vi "4Pi 4Pi Modes - Mode Scan Engine.vi"() -> ()   [LabVIEW 2016]
uses:
  4Pi 4Pi Modes - Controls/4Pi 4Pi Modes - Mode Scan - Gaussian Initial Guesses.ctl
  4Pi 4Pi Modes - Controls/4Pi 4Pi Modes - Mode Scan - Metric Fit Type.ctl
  4Pi 4Pi Modes - Controls/4Pi 4Pi Modes - Mode Scan - Scan Settings.ctl
  4Pi 4Pi Modes - Controls/4Pi 4Pi Modes - Mode Scan - Metric.ctl
  4Pi 4Pi Modes - Controls/4Pi 4Pi Modes - Mode Scan - Threshold Mean Limits.ctl
  4Pi 4Pi Modes - Controls/4Pi 4Pi Modes - Mode Scan - Image Type.ctl
  4Pi 4Pi Modes - Controls/4Pi 4Pi Modes - Mode Scan - Blink Scan Settings.ctl
  4Pi 4Pi Modes - Controls/4Pi 4Pi Modes - Mode Scan - Blink Analysis Type.ctl
  <vilib>/vision/Image Controls.llb/IMAQ Image.ctl
  Hardware Configuration/Hardware Configuration Controls/Device Type.ctl
  Hardware Configuration/Hardware Configuration Controls/Device Function.ctl
  <vilib>/Utility/miscctls.llb/LVPointTypeDef.ctl
  4Pi 4Pi Modes - Controls/4Pi 4Pi Modes - Mode Scan - Last Used Data Type.ctl
  4Pi 4Pi Modes - Controls/4Pi 4Pi Modes - Mode Scan - Notifier Type.ctl
  4Pi 4Pi Modes - Controls/4Pi 4Pi Modes - Mode Scan - Scan Actions.ctl
  4Pi 4Pi Modes - Controls/4Pi 4Pi Modes - Standard Action.ctl
  4Pi 4Pi Modes - Controls/4Pi 4Pi Modes - Standard Counter Action.ctl
  <vilib>/Analysis/6fits.llb/Curve Fitting Criteria.ctl
  <vilib>/Analysis/baseanly.llb/Mean (DBL).vi
  <vilib>/Analysis/NI_AALBase.lvlib
  <vilib>/Analysis/NI_AALPro.lvlib
  <vilib>/gmath/NI_Gmath.lvlib
  <resource>/objmgr/IMAQImage.rc
panel:
  in  "Calling VI Ref":refnum<vi>
  in  "Main Tab":enum32{"Scan Modes", "Settings"}(tab)
  in  "Fit Data":bool
  in  "Apply":bool
  in  "Get Image":bool
  in  "Current Mode":i32(ring) items=["1", "2", "3", "4", "5", "6", "7", "8", "9", "10", "11", "12", "13", "14", "15", "16", "17", "18", "19", "20", "21", "22", "23", "24", "25", "26", "27", "28", "29", "30", "31", "32", "33", "34", "35", "36", "37", "38", "39", "40", "41", "42", "43", "44", "45", "46", "47", "48", "49", "50", "51", "52", "53", "54", "55", "56", "57", "58", "59", "60", "61", "62", "63", "64", "65", "66", "67", "68", "69", "70", "71", "72", "73", "74", "75", "76", "77", "78", "79", "80", "81", "82", "83", "84", "85", "86", "87", "88", "89", "90", "91", "92", "93", "94", "95", "96", "97", "98", "99", "100", "101", "102", "103", "104", "105", "106", "107", "108", "109", "110", "111", "112", "113", "114", "115", "116", "117", "118", "119", "120", "121", "122", "123", "124", "125", "126", "127", "128", "129", "130", "131", "132", "133", "134", "135", "136", "137", "138", "139", "140"]
  in  "Scan Mode":bool
  in  "Scan Next Mode":bool
  in  "Auto Scan Modes":bool
  out "Metric":cluster{dbl[], dbl[]}[](graph)
  out "AO Image Display":T1(plugin-control)
  in  "Gaussian Initial Guesses":T2={"Amplitude"=2500.0, "Center Position"=0.0, "Width (Sigma)"=200.0, "Offset"=500.0, "User Guesses"=TRUE}
  in  "DM Scan Settings":T3={"Frame Delay"=1, "Frame Accumulations"=2, "Number of Steps"=8, "Step Size (nm)"=80}
  in  "Image Type":T4 items=["Full Image", "ROI", "Blinks"]
  in  "Image Selection":i32(ring) items=["Quad 01", "Quad 02", "Quad 03", "Quad 04"]
  in  "Metric":T5=1 items=["Max Intensity", "No Zero Mean", "Threshold Mean", "Mean"]
  in  "Metric Fit Type":T6 items=["Guassian", "Quadratic"]
  in  "Threshold Mean Limits":T7={"Upper Limit"=10000.0, "Lower Limit"=0.0}
  in  "Blink Scan Settings":T8={"Blink Analysis Type"=1, "Blink ROI Box Width"=0, "Blink Threshold"=0.0} {"Blink Analysis Type" items=["Mean Intensity", "2D Fit Intensity"]}
  in  "Exit":bool
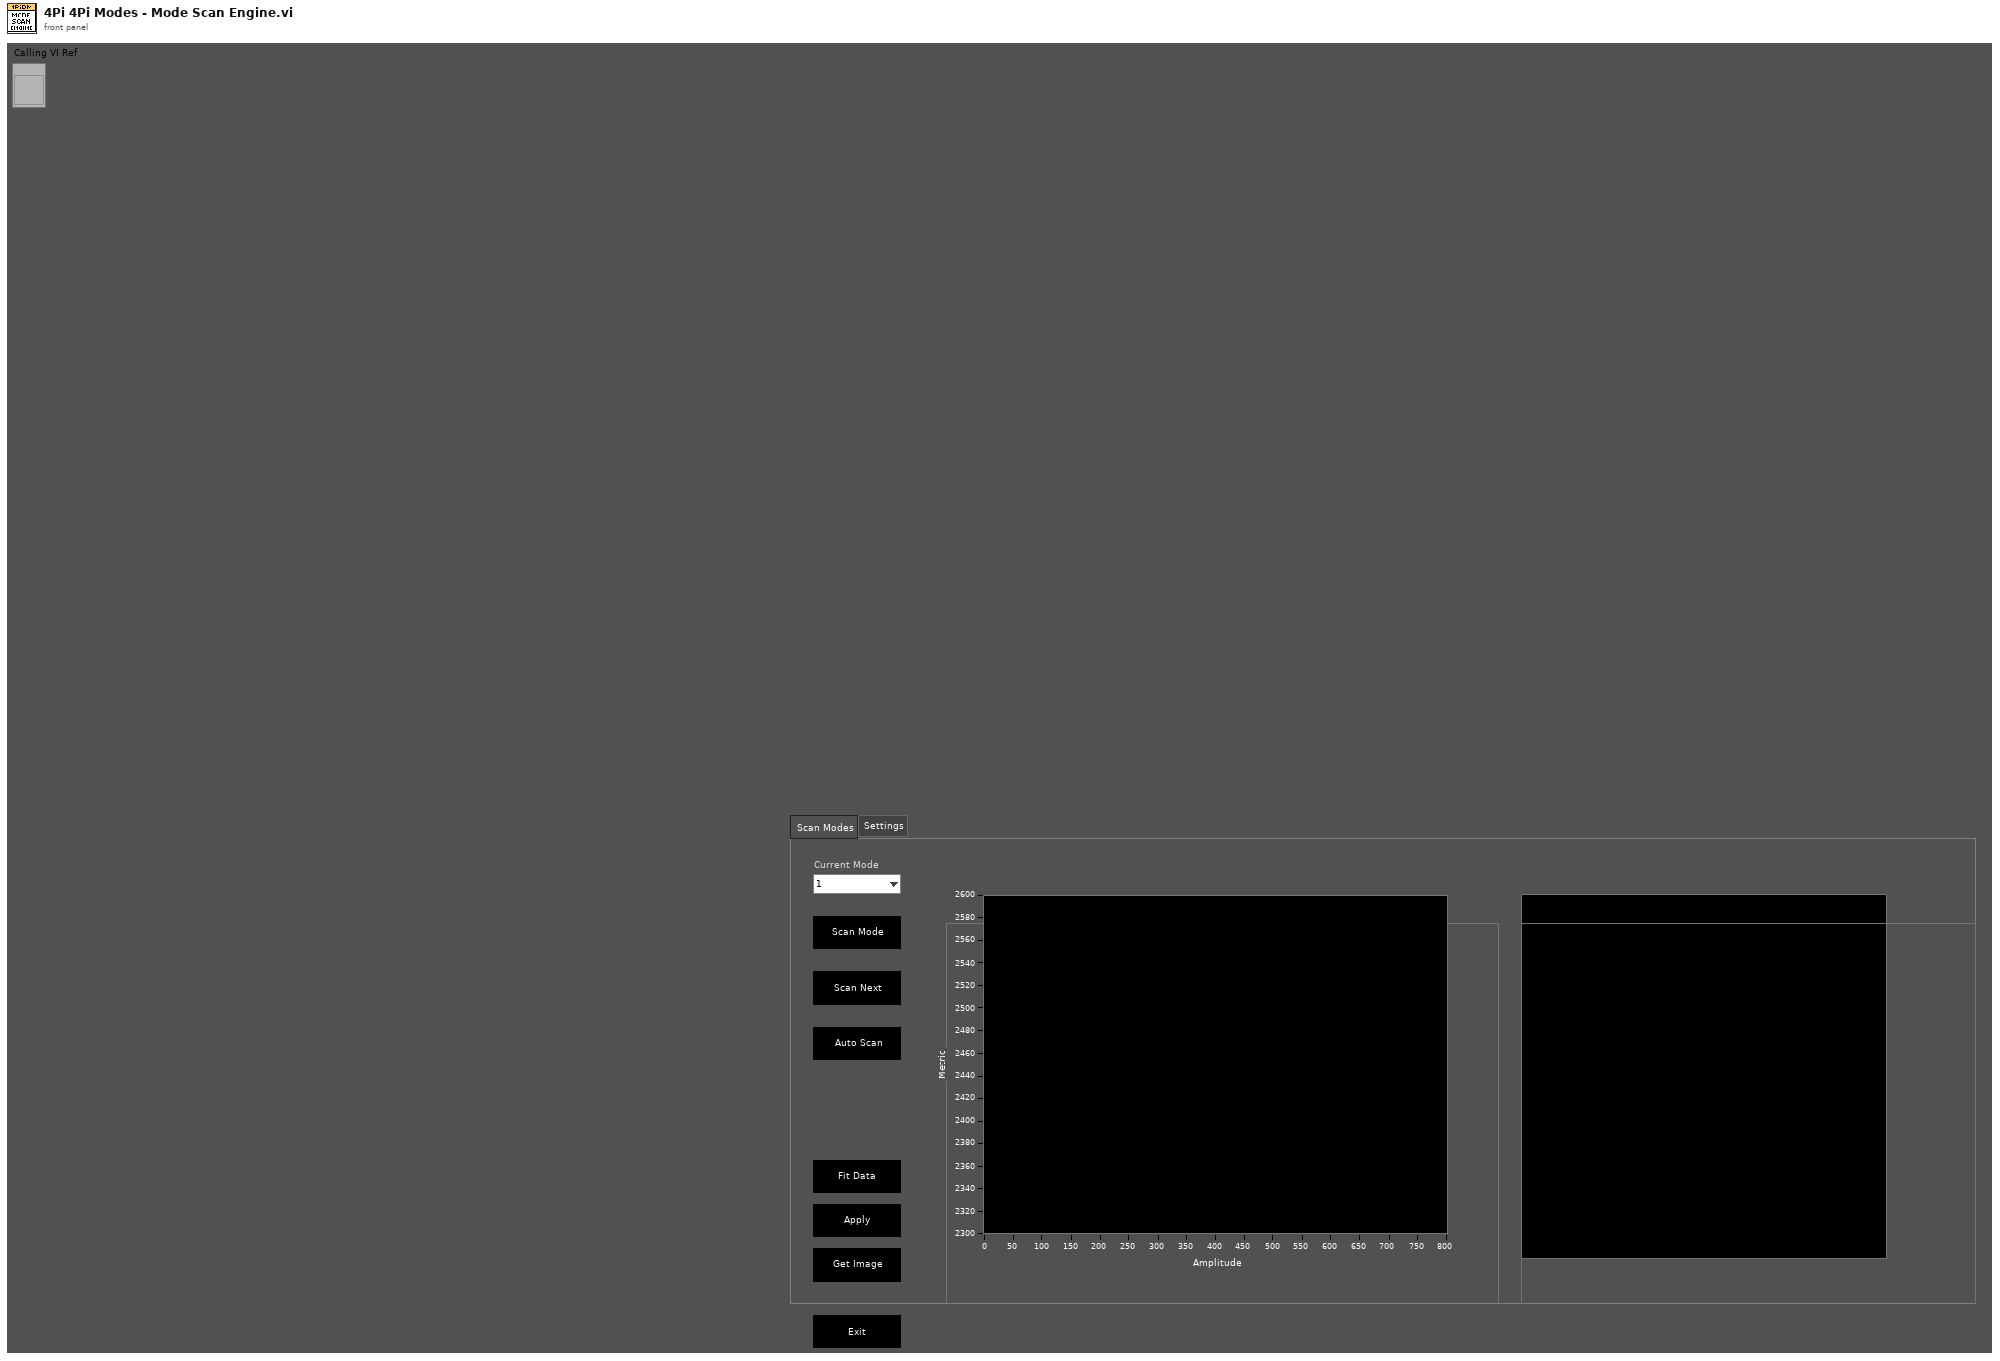
[diagram p1: front panel]
types:
  T1 = typedef "IMAQ Image.ctl" = refnum<image>
  T2 = typedef "4Pi 4Pi Modes - Mode Scan - Gaussian Initial Guesses.ctl" = cluster{"Amplitude":dbl, "Center Position":dbl, "Width (Sigma)":dbl, "Offset":dbl, "User Guesses":bool}
  T3 = typedef "4Pi 4Pi Modes - Mode Scan - Scan Settings.ctl" = cluster{"Frame Delay":u32, "Frame Accumulations":u16, "Number of Steps":u16, "Step Size (nm)":u16}
  T4 = typedef "4Pi 4Pi Modes - Mode Scan - Image Type.ctl" = u16
  T5 = typedef "4Pi 4Pi Modes - Mode Scan - Metric.ctl" = u16
  T6 = typedef "4Pi 4Pi Modes - Mode Scan - Metric Fit Type.ctl" = u16
  T7 = typedef "4Pi 4Pi Modes - Mode Scan - Threshold Mean Limits.ctl" = cluster{"Upper Limit":dbl, "Lower Limit":dbl}
  T8 = typedef "4Pi 4Pi Modes - Mode Scan - Blink Scan Settings.ctl" = cluster{"Blink Analysis Type":T9, "Blink ROI Box Width":u8, "Blink Threshold":sgl}
  T9 = typedef "4Pi 4Pi Modes - Mode Scan - Blink Analysis Type.ctl" = u16
  T10 = typedef "Image Type" = u32
  T11 = enum8{"Enabled", "Disabled", "Disabled and Grayed Out"}
  T12 = typedef "4Pi 4Pi Modes - Mode Scan - Scan Actions.ctl" = enum16{"Scan Mode", "Fit Data", "Scan Next Mode", "Update Mode Amount", "Get Image", "Compute Metric", "Update Counter", "Apply Correction", "Exit", "Quit"}
  T13 = typedef "4Pi 4Pi Modes - Mode Scan - Notifier Type.ctl" = cluster{"Action":T12, "Image Ref":T1, "Image Type":T4, "Fit Type":T6, "Metric":T5, "Scan Running?":bool, "DM Scan Settings":T3, "Threshold Mean Limits":T7, "Gaussian Initial Guesses":T2, "Blink Scan Settings":T8}
  T14 = typedef "4Pi 4Pi Modes - Mode Scan - Last Used Data Type.ctl" = cluster{"Image Ref Index":i32, "Image Type":T4, "Fit Type":T6, "Metric":T5, "DM Scan Settings":T3, "Threshold Mean Limits":T7, "Gaussian Initial Guesses":T2, "Blink Scan Settings":T8}
  T15 = enum16{"Always On", "Always Off", "Off While Running"}
  T16 = typedef "LVPointTypeDef.ctl" = cluster{"Horizontal":i16, "Vertical":i16}
  T17 = typedef "Device Function.ctl" = enum16{"Primary", "Secondary", "Overview", "Wide Field Drift Correction", "642 nm Excitation", "560 nm Excitation", "940 nm Excitation", "546 nm Excitation", "488 nm Excitation", "405 nm Excitation", "Objective Drift Correction", "4Pi Objective Lock", "Objective XY", "Objective Z", "Sample XY", "Sample Coarse Z", "Sample Z", "4Pi Lower", "4Pi Upper", "Mojo", "Adj Cavity", "Line Scanning", "Alert"}
  T18 = typedef "Device Type.ctl" = enum16{"AOTF", "Camera", "Deformable Mirror", "Laser", "Shutter", "Stage", "Waveform", "FPGA", "Email"}
  T19 = typedef "LVRectTypeDef.ctl" = cluster{"Left":i16, "Top":i16, "Right":i16, "Bottom":i16}
  T20 = typedef "LVBoundsTypeDef.ctl" = cluster{"Width":u32, "Height":u32}
  T21 = typedef "4Pi 4Pi Modes - Standard Action.ctl" = enum16{"Read", "Write"}
  T22 = typedef "4Pi 4Pi Modes - Standard Counter Action.ctl" = enum16{"Initialize", "Update Count", "Get Count"}
  T23 = cluster{"initial amplitude":dbl, "initial center":dbl, "initial standard deviation":dbl, "offset":dbl}
  T24 = cluster{"amp min":dbl, "amp max":dbl, "center min":dbl, "center max":dbl, "deviation min":dbl, "deviation max":dbl, "offset min":dbl, "offset max":dbl}
  T25 = enum16{"Linear", "Polynomial", "Exponential", "Power"}
  T26 = cluster{"Global Rectangle":i32[], "Contours":cluster{"Contour Type":u32, "ROI Type":u32, "Points":i32[]}[]}
  T27 = cluster{"Amplitude Out":dbl[], "Metric Out":dbl[]}
  T28 = cluster{"initial amplitude":dbl, "Numeric":dbl, "initial standard deviation":dbl, "offset":dbl}
  T29 = typedef "NI_AALPro.lvlib/Curve Fitting Criteria.ctl" = u16
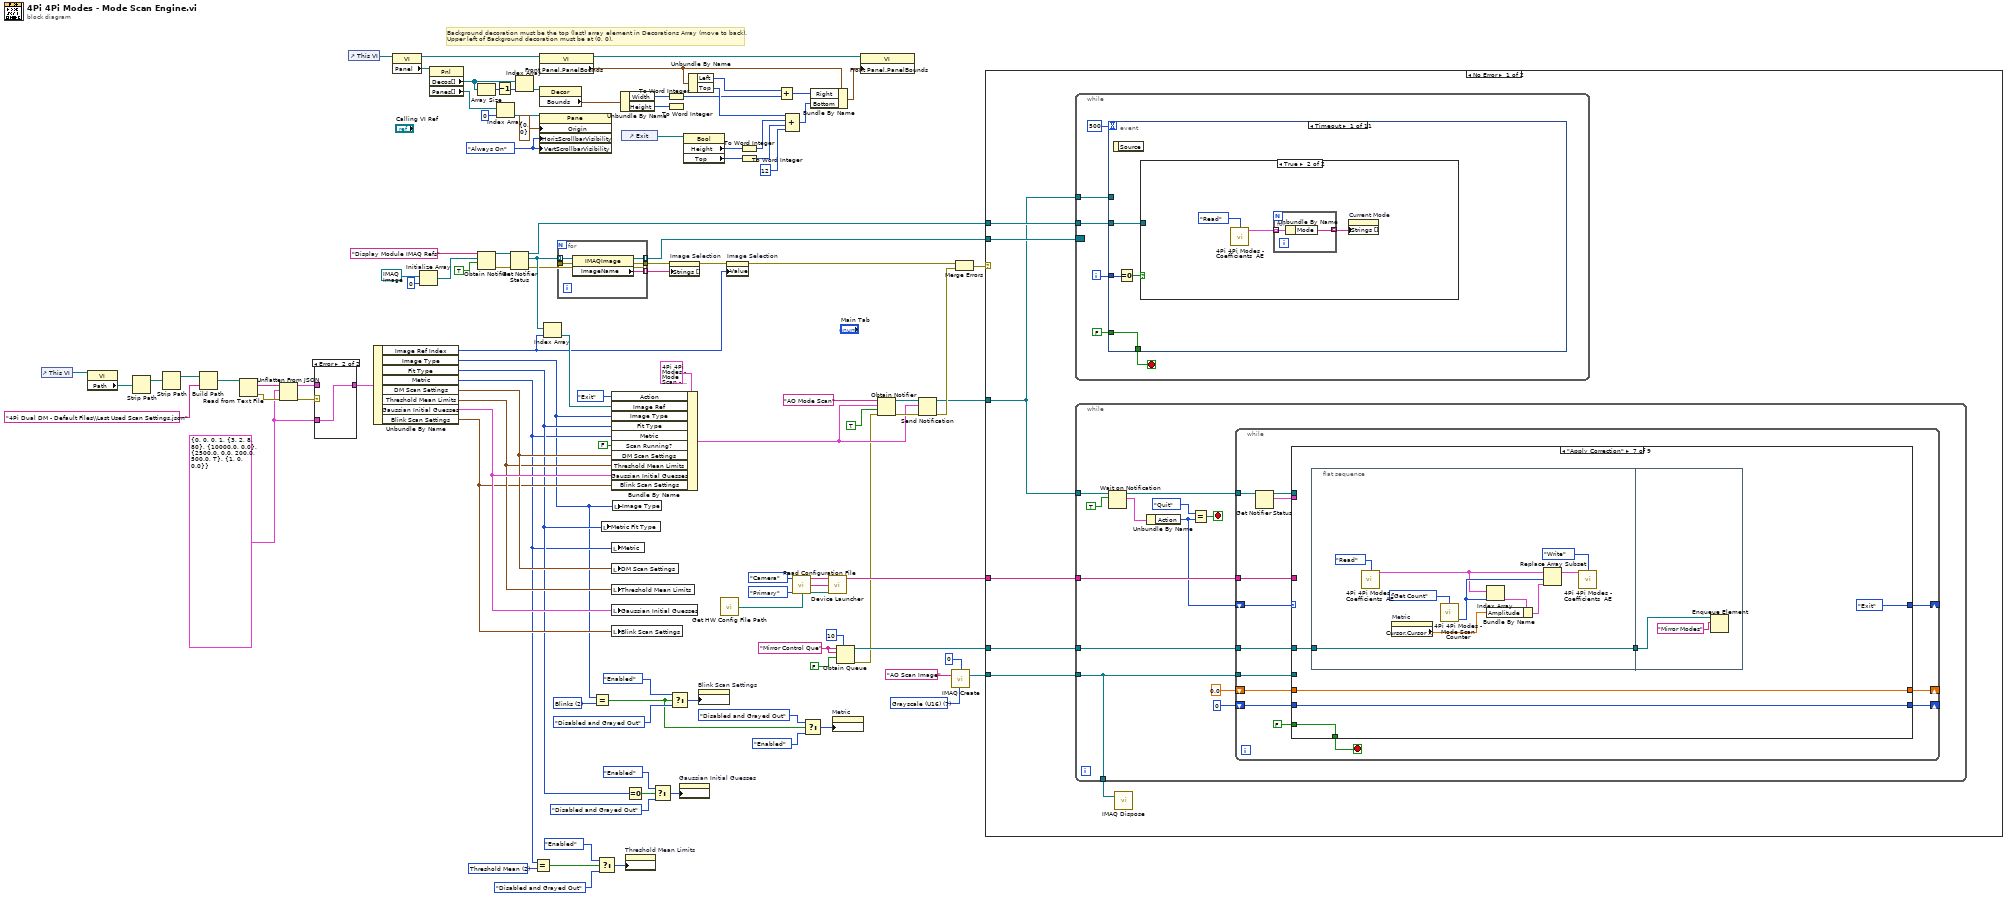
[diagram p0: block diagram]
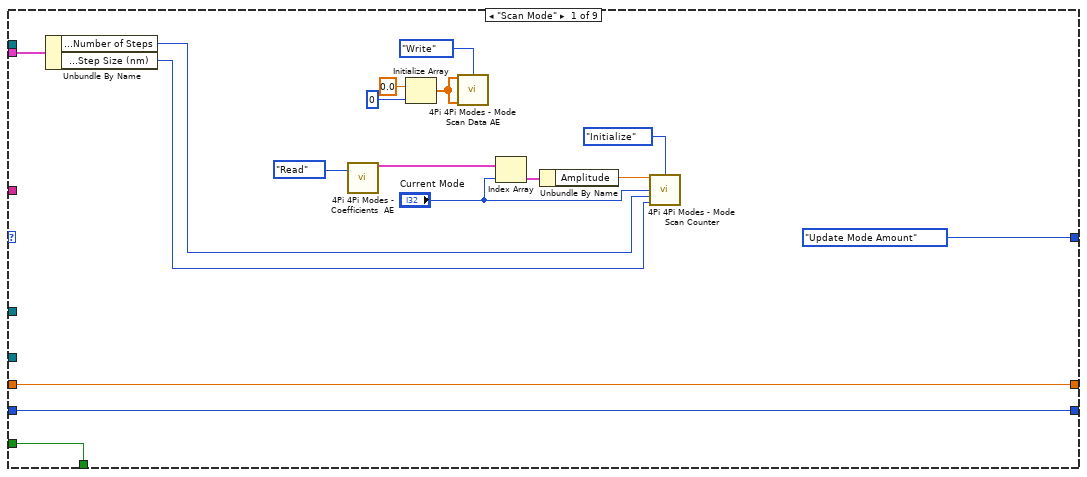
[diagram p2: hidden frame]
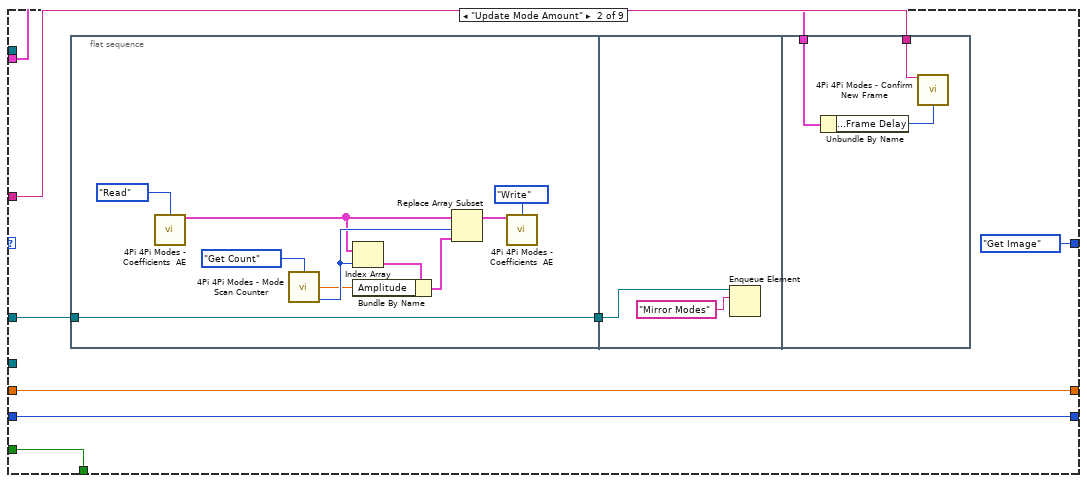
[diagram p3: hidden frame]
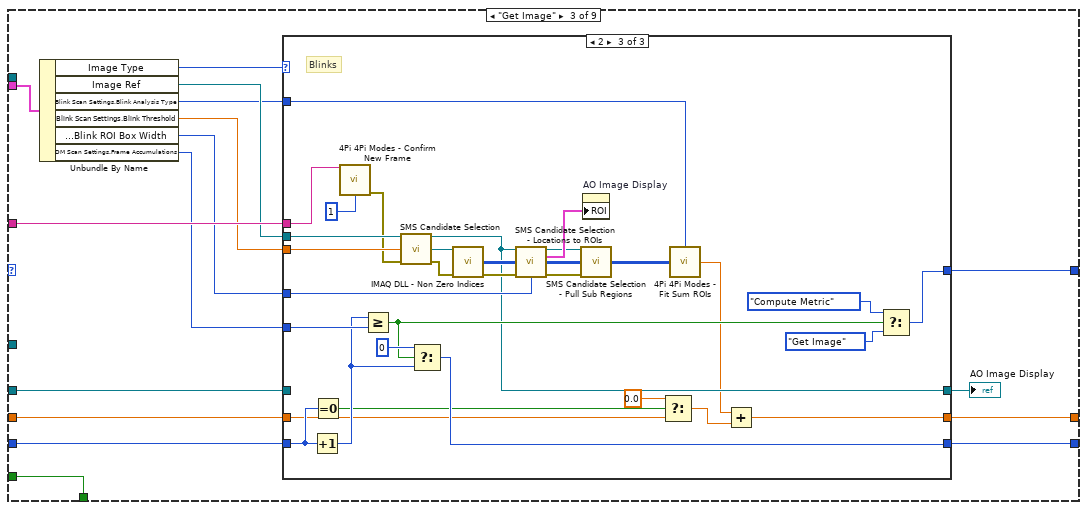
[diagram p4: hidden frame]
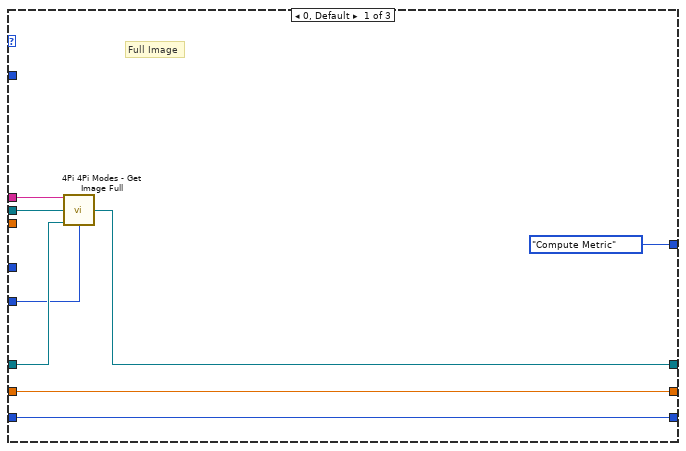
[diagram p5: hidden frame]
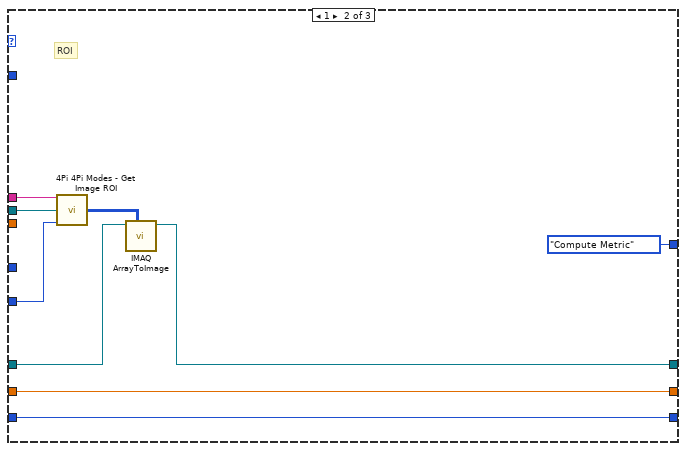
[diagram p6: hidden frame]
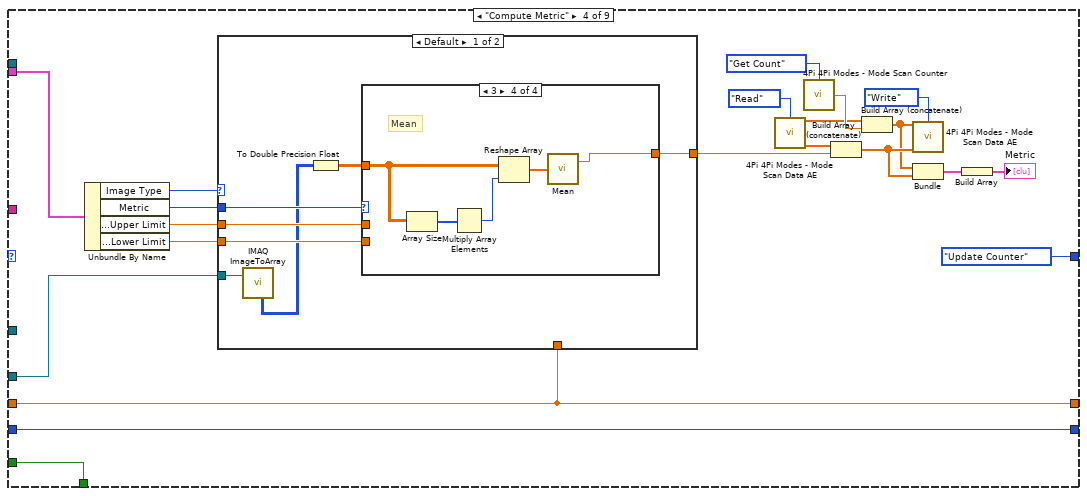
[diagram p7: hidden frame]
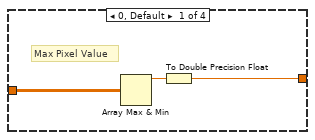
[diagram p8: hidden frame]
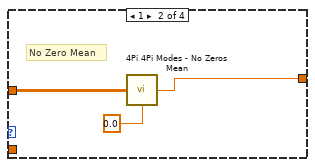
[diagram p9: hidden frame]
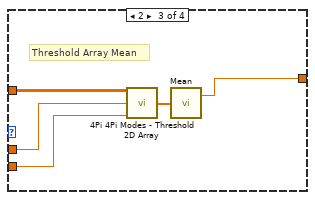
[diagram p10: hidden frame]
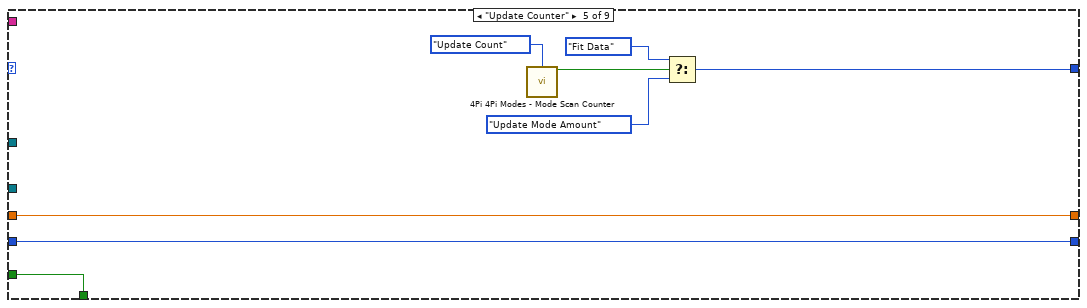
[diagram p12: hidden frame]
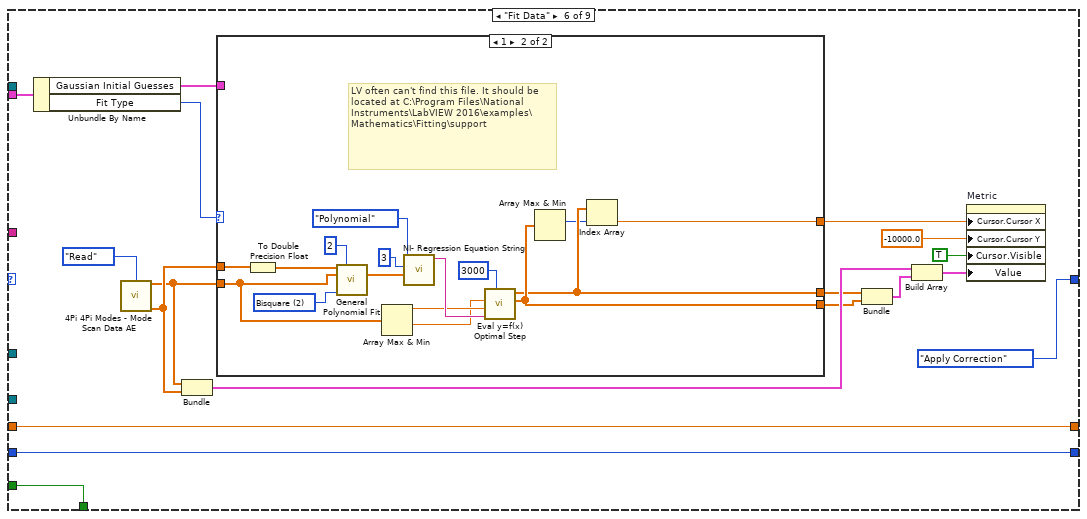
[diagram p13: hidden frame]
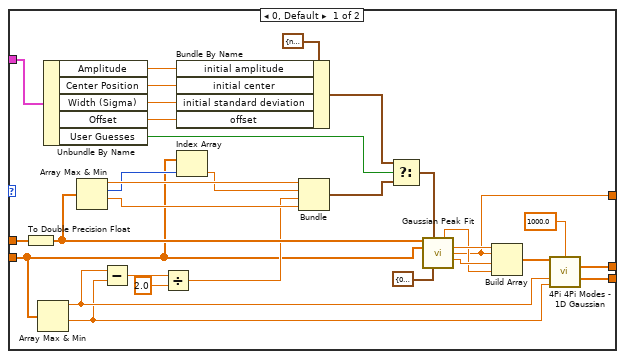
[diagram p14: hidden frame]
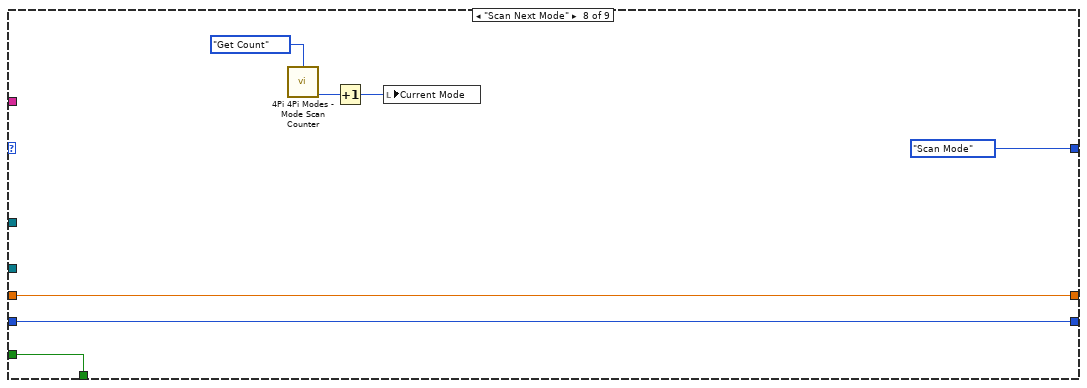
[diagram p15: hidden frame]
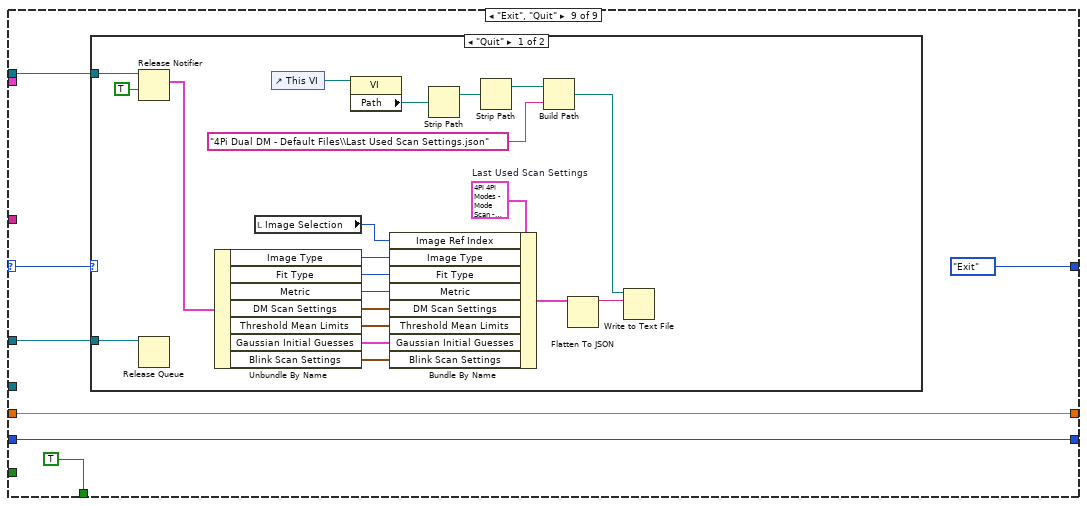
[diagram p16: hidden frame]
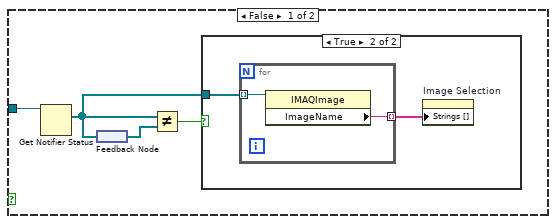
[diagram p18: hidden frame]
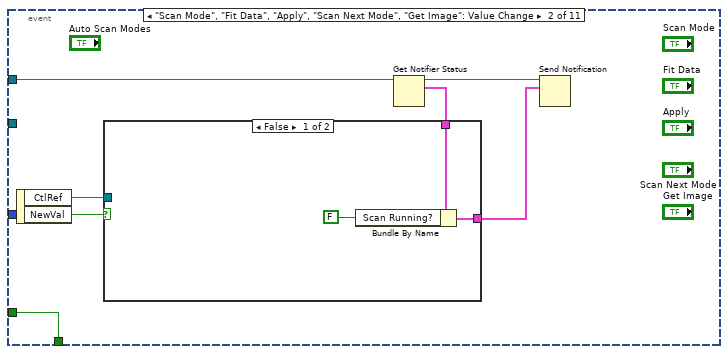
[diagram p20: hidden frame]
diagram:
  w2 = T10 7 items=["Grayscale (U8)", "Grayscale (I16)", "Grayscale (SGL)", "Complex (CSG)", "RGB (U32)", "HSL (U32)", "RGB (U64)", "Grayscale (U16)"] ("Image Type")
  w12 = T4 2 items=["Full Image", "ROI", "Blinks"] ("y")
  w15 = T5 2 items=["Max Intensity", "No Zero Mean", "Threshold Mean", "Mean"] ("y")
  w45 = T14 {"Image Ref Index"=0, "Image Type"=0, "Fit Type"=0, "Metric"=1, "DM Scan Settings"={"Frame Delay"=3, "Frame Accumulations"=2, "Number of Steps"=8, "Step Size (nm)"=80}, "Threshold Mean Limits"={"Upper Limit"=10000.0, "Lower Limit"=0.0}, "Gaussian Initial Guesses"={"Amplitude"=2500.0, "Center Position"=0.0, "Width (Sigma)"=200.0, "Offset"=500.0, "User Guesses"=TRUE}, "Blink Scan Settings"={"Blink Analysis Type"=1, "Blink ROI Box Width"=0, "Blink Threshold"=0.0}} ("Mode Scan Notifier Type")
  w76 = T15."Always On" ("Vertical Scrollbar Visibility")
  w109 = "Mirror Control Que" ("name (unnamed)")
  # "Background decoration must be the top (last) array element in Decorations Array (move to back).\nUpper left of Background decoration must be at (0, 0)."
  n1 = control-ref of="This VI"() -> (w58:refnum<vi>)
  n2 = property class="VI"(reference=w58) -> ("Path"=w57:path)  [unwired: 1 in, 2 out]
  n3 = Strip Path(path=w57) -> (stripped path=w56:path)  [unwired: 1 out]
  n4 = Strip Path(path=w56) -> (stripped path=w55:path)  [unwired: 1 out]
  n5 = Build Path(base path=w55, name or relative path="4Pi Dual DM - Default Files\\Last Used Scan Settings.json") -> (appended path=w52:path)
  n6 = Read from Text File(file (use dialog)=w52) -> (text=w53:string, error out=w51:errorcluster)  [unwired: 3 in, 2 out]
  n7 = Unflatten From JSON(JSON string=w53, type and defaults=w45, error in (no error)=w51) -> (value=w44:T14, error out=w50:errorcluster)  [unwired: 4 in]
  n8 = case shown="Error" w50 {
    tunnel: w45 -> [_ w111]
    tunnel: w44 -> [w110 _]
    tunnel: [w110 w111] -> w41
    frame No Error {
    }
    frame Error {
    }
  }
  n9 = control-ref of="This VI"() -> (w68:refnum<vi>)
  n10 = Unbundle By Name(w41) -> ("Image Ref Index"=w39:i32, "Image Type"=w9:T4, "Fit Type"=w24:T6, "Metric"=w14:T5, "DM Scan Settings"=w27:T3, "Threshold Mean Limits"=w26:T7, "Gaussian Initial Guesses"=w28:T2, "Blink Scan Settings"=w25:T8)
  n11 = property class="VI"(reference=w68) -> (reference out=w77:refnum<vi>, "Panel"=w69:refnum<vi>)  [unwired: 1 in, 1 out]
  n12 = Initialize Array(T1 refnum ("New Image"), 0 ("dimension size")) -> (w102:T1[])
  n13 = property class="Pnl"(reference=w69) -> ("Decos[]"=w67:refnum<vi>[], "Panes[]"=w73:refnum<vi>[])  [unwired: 1 in, 2 out]
  n14 = Obtain Notifier(name (unnamed)="Display Module IMAQ Refs", notification data type=w102, create if not found? (T)=TRUE) -> (notifier out=w101:refnum<notifier>, error out=w63:errorcluster)  [unwired: 1 in, 1 out]
  n15 = Array Size(array=w67) -> (size(s)=w65:i32)
  n16 = Decrement(x=w65) -> (x-1=w66:i32)
  n17 = Index Array(array=w73, index=0) -> (element=w72:refnum<vi>)
  n18 = Get Notifier Status(notifier=w101, error in (no error)=w63) -> (notifier out=w34:refnum<notifier>, current notification=w64:T1[], error out=w62:errorcluster)  [unwired: 2 out]
  n19 = Index Array(array=w67, index=w66) -> (element=w75:refnum<vi>)
  n20 = Equal?(x=w14, y=w15) -> (x = y?=w16:bool)
  n21 = property class="VI"(reference=w77) -> (reference out=w79:refnum<vi>, "Front Panel.PanelBounds"=w80:T19)  [unwired: 1 in, 1 out]
  n22 = property class="Decor"(reference=w75) -> ("Bounds"=w78:T20)  [unwired: 1 in, 2 out]
  n23 = property class="Pane"(reference=w72, "Origin"=T16 {"Horizontal"=0, "Vertical"=0}, "HorizScrollbarVisibility"=w76, "VertScrollbarVisibility"=w76) -> ()  [unwired: 1 in, 2 out]
  n24 = Index Array(array=w64, index=w39) -> (element=w40:T1)
  n25 = for {
    tunnel: w64 -> [w116] mode=indexing
    tunnel: [w115] -> w61 mode=indexing
    tunnel: [w114] -> w60
    tunnel: [w113] -> w33 mode=indexing
    tunnel: w62 -> [w112]
    n26 = property class="IMAQImage"(reference=w116, error in=w112) -> (reference out=w113:T1, error out=w114:errorcluster, "ImageName"=w115:string)
  }
  n27 = Equal?(x=w9, y=w12) -> (x = y?=w5:bool)
  n28 = Select(t=T11."Enabled" ("Disabled"), s=w16, f=T11."Disabled and Grayed Out" ("Disabled")) -> (s? t:f=w19:T11)
  n29 = local write "Metric Fit Type"(w24) -> ()
  n30 = Bundle By Name(cluster=T13 {"Action"=enum."Scan Mode", "Image Ref"=refnum, "Image Type"=0, "Fit Type"=0, "Metric"=1, "Scan Running?"=FALSE, "DM Scan Settings"={"Frame Delay"=1, "Frame Accumulations"=2, "Number of Steps"=8, "Step Size (nm)"=80}, "Threshold Mean Limits"={"Upper Limit"=10000.0, "Lower Limit"=0.0}, "Gaussian Initial Guesses"={"Amplitude"=2500.0, "Center Position"=0.0, "Width (Sigma)"=200.0, "Offset"=500.0, "User Guesses"=TRUE}, "Blink Scan Settings"={"Blink Analysis Type"=1, "Blink ROI Box Width"=0, "Blink Threshold"=0.0}} ("Mode Scan Notifier Type"), "Action"=4Pi_4Pi_Modes_-_Mode_Scan_-_Scan_Actions."Exit", "Image Ref"=w40, "Image Type"=w9, "Fit Type"=w24, "Metric"=w14, "Scan Running?"=FALSE, "DM Scan Settings"=w27, "Threshold Mean Limits"=w26, "Gaussian Initial Guesses"=w28, "Blink Scan Settings"=w25) -> (w37:T13)
  n31 = local write "Metric"(w14) -> ()
  n32 = local write "DM Scan Settings"(w27) -> ()
  n33 = local write "Threshold Mean Limits"(w26) -> ()
  n34 = local write "Gaussian Initial Guesses"(w28) -> ()
  n35 = local write "Blink Scan Settings"(w25) -> ()
  n36 = local write "Image Type"(w9) -> ()
  n37 = Unbundle By Name(w78) -> ("Width"=w83:u32, "Height"=w86:u32)
  n38 = control-ref of="Exit"() -> (w70:refnum<vi>)
  n39 = property on="Threshold Mean Limits" class="Clust (strict)"("DisabledEnum"=w19) -> ()  [unwired: 2 in, 2 out]
  n40 = Equal To 0?(x=w24) -> (x = 0?=w23:bool)
  n41 = Select(t=T11."Enabled" ("Disabled"), s=w23, f=T11."Disabled and Grayed Out" ("Disabled")) -> (s? t:f=w20:T11)
  n42 = To Word Integer(number=w83) -> (16bit integer=w85:i16)
  n43 = To Word Integer(number=w86) -> ()  [unwired: 1 out]
  n44 = property on="Image Selection" class="Ring (strict)"(error in=w60, "Strings []"=w61) -> (error out=w59:errorcluster)  [unwired: 1 in, 1 out]
  n45 = Select(t=T11."Enabled" ("Disabled"), s=w5, f=T11."Disabled and Grayed Out" ("Disabled")) -> (s? t:f=w13:T11)
  n46 = property on="Gaussian Initial Guesses" class="Clust (strict)"("DisabledEnum"=w20) -> ()  [unwired: 2 in, 2 out]
  n47 = property class="Bool"(reference=w70) -> ("Height"=w88:u32, "Top"=w89:i32)  [unwired: 1 in, 2 out]
  n48 = Unbundle By Name(w80) -> ("Left"=w82:i16, "Top"=w93:i16)
  n49 = property on="Blink Scan Settings" class="Clust (strict)"("DisabledEnum"=w13) -> ()  [unwired: 2 in, 2 out]
  n50 = call "Get HW Config File Path.vi"() -> ("File Path"=w95:path)  [unwired: 14 in, 1 out]
  n51 = property on="Image Selection" class="Ring (strict)"(error in=w59, "Value"=w39) -> (error out=w32:errorcluster)  [unwired: 1 in, 1 out]
  n52 = To Word Integer(number=w88) -> (16bit integer=w91:i16)
  n53 = To Word Integer(number=w89) -> (16bit integer=w92:i16)
  n54 = Add(x=w82, y=w85) -> (x+y=w84:i16)
  n55 = Compound Arithmetic op=ADD(w93, w91, w92, i16 12 ("y")) -> (w87:i16)
  n56 = call "Read Configuration File.vi"("Device Type"=Device_Type."Camera", "Device Function"=Device_Function."Primary", "Config File Path"=w95) -> ("Unique Notifier Name"=w96:string, "Device Ports/IDs/Channels"=w98:string[], "Device Engine Path"=w97:path)  [unwired: 9 in, 1 out]
  n57 = Select(t=T11."Disabled and Grayed Out" ("Disabled"), s=w5, f=T11."Enabled" ("Disabled")) -> (s? t:f=w6:T11)
  n58 = Bundle By Name(cluster=w80, "Right"=w84, "Bottom"=w87) -> (w81:T19)
  n59 = call "Device Launcher.vi"("Notifier Name"=w96, "Device Ports/IDs/Channels"=w98, "Device Engine Path"=w97) -> ("Notifier Name"=w94:string)  [unwired: 11 in, 1 out]
  n60 = property on="Metric" class="Ring (strict)"("DisabledEnum"=w6) -> ()  [unwired: 2 in, 2 out]
  n61 = Obtain Queue(max queue size (-1, unlimited)=10, name (unnamed)=w109, element data type=w109, create if not found? (T)=FALSE) -> (queue out=w107:refnum<queue>, error out=w35:errorcluster)  [unwired: 1 in, 1 out]
  n62 = property class="VI"(reference=w79, "Front Panel.PanelBounds"=w81) -> ()  [unwired: 1 in, 2 out]
  n63 = Obtain Notifier(name (unnamed)="AO Mode Scan", notification data type=w37, create if not found? (T)=TRUE, error in (no error)=w35) -> (notifier out=w46:refnum<notifier>, error out=w47:errorcluster)  [unwired: 1 out]
  n64 = Send Notification(notification=w37, notifier=w46, error in (no error)=w47) -> (notifier out=w29:refnum<notifier>, error out=w31:errorcluster)
  n65 = call "IMAQ Create"("Border Size"=0, "Image Name"="AO Scan Image", "Image Type"=w2) -> ("New Image"=w1:T1)  [unwired: 2 in, 1 out]
  n66 = Merge Errors(w32, w31) -> (w30:errorcluster)
  n67 = case shown="No Error" w30 {
    tunnel: w107 -> [w123 w554]
    tunnel: w94 -> [w122 _]
    tunnel: w34 -> [w121 w552]
    tunnel: w33 -> [w120 _]
    tunnel: w29 -> [w119 w553]
    tunnel: w1 -> [w118 w555]
    frame No Error {
      n68 = while {
        tunnel: w121 -> [w429]
        border: w120 -> [_]
        tunnel: w119 -> [w428]
        i -> [w431]
        stop <- w426 stop-if-true
        n69 = event shown="[0] Timeout" {
          selector: _ -> [_ _ _ _ _ _ _ _ _ _ _]
          dyn-events: _ -> [_ _ _ _ _ _ _ _ _ _ _]
          timeout: 500 -> [_ _ _ _ _ _ _ _ _ _ _]
          tunnel: w431 -> [w435 _ _ _ _ _ _ _ _ _ _]
          tunnel: w429 -> [w433 _ w479 _ _ _ _ _ _ _ w551]
          tunnel: w428 -> [_ w454 w478 w487 w500 w515 w523 w530 w537 w544 w549]
          tunnel: [w432 w450 w470 w480 w501 w516 w517 w524 w531 w538 TRUE] -> w426
          tunnel: FALSE -> [w432 w450 w470 w480 w501 w516 w517 w524 w531 w538 _]
          event Timeout {
            n70 = event-data() -> ()  [unwired: 1 in, 1 out]
            n71 = Equal To 0?(x=w435) -> (x = 0?=w434:bool)
            n72 = case shown="True" w434 {
              tunnel: w433 -> [w439 _]
              frame False {
                n73 = Get Notifier Status(notifier=w439) -> (current notification=w436:T1[])  [unwired: 1 in, 4 out]
                n74 = feedback-in #1(w436) -> ()
                n75 = feedback #1() -> (w438:T1[])
                n76 = Not Equal?(x=w436, y=w438) -> (x != y?=w437:bool)
                n77 = case shown="True" w437 {
                  tunnel: w436 -> [_ w441]
                  frame False {
                  }
                  frame True {
                    n78 = for {
                      tunnel: w441 -> [w443] mode=indexing
                      tunnel: [w442] -> w440 mode=indexing
                      n79 = property class="IMAQImage"(reference=w443) -> ("ImageName"=w442:string)  [unwired: 1 in, 2 out]
                    }
                    n80 = property on="Image Selection" class="Ring (strict)"("Strings []"=w440) -> ()  [unwired: 2 in, 2 out]
                  }
                }
              }
              frame True {
                n81 = call "4Pi 4Pi Modes - Coefficients  AE.vi"("Action"=4Pi_4Pi_Modes_-_Standard_Action."Read") -> ("Coefficients Out"=w445:cluster{"Mode":string, "Amplitude":dbl}[])  [unwired: 14 in]
                n82 = for {
                  tunnel: [w448] -> w444 mode=indexing
                  tunnel: w445 -> [w447] mode=indexing
                  n83 = Unbundle By Name(w447) -> ("Mode"=w448:string)
                }
                n84 = property on="Current Mode" class="Ring (strict)"("Strings []"=w444) -> ()  [unwired: 2 in, 2 out]
              }
            }
          }
          event "Scan Mode", "Fit Data", "Apply", "Scan Next Mode", "Get Image": Value Change {
            n85 = event-data() -> ("CtlRef"=w455:refnum<vi>, "NewVal"=w449:bool)  [unwired: 1 in]
            n86 = Get Notifier Status(notifier=w454) -> (notifier out=w453:refnum<notifier>, current notification=w452:T13)  [unwired: 1 in, 3 out]
            n87 = case shown="False" w449 {
              tunnel: w455 -> [_ w463]
              tunnel: w452 -> [w458 w462]
              tunnel: [w457 w461] -> w451
              frame False {
                n88 = Bundle By Name(cluster=w458, "Scan Running?"=FALSE) -> (w457:T13)
              }
              frame True {
                n89 = property class="Bool"(reference=w463) -> ("Label.Text"=w460:string)  [unwired: 1 in, 2 out]
                n90 = case shown="\"Apply\"" w460 {
                  tunnel: [4Pi_4Pi_Modes_-_Mode_Scan_-_Scan_Actions."Scan Mode" ("Action") 4Pi_4Pi_Modes_-_Mode_Scan_-_Scan_Actions."Scan Mode" ("Action") 4Pi_4Pi_Modes_-_Mode_Scan_-_Scan_Actions."Fit Data" ("Action") 4Pi_4Pi_Modes_-_Mode_Scan_-_Scan_Actions."Apply Correction" ("Action") 4Pi_4Pi_Modes_-_Mode_Scan_-_Scan_Actions."Scan Next Mode" ("Action") 4Pi_4Pi_Modes_-_Mode_Scan_-_Scan_Actions."Get Image" ("Action")] -> w459
                  frame Default {
                  }
                  frame "Scan Mode" {
                  }
                  frame "Fit Data" {
                  }
                  frame "Apply" {
                  }
                  frame "Scan Next Mode" {
                  }
                  frame "Get Image" {
                  }
                }
                n91 = Bundle By Name(cluster=w462, "Action"=w459) -> (w461:T13)
              }
            }
            n92 = Send Notification(notification=w451, notifier=w453) -> ()  [unwired: 1 in, 2 out]
          }
          event "Image Selection": Value Change {
            n93 = event-data() -> ("NewVal"=w471:i32)  [unwired: 1 in]
            n94 = Get Notifier Status(notifier=w479) -> (current notification=w477:T1[])  [unwired: 1 in, 4 out]
            n95 = Index Array(array=w477, index=w471) -> (element=w475:T1)
            n96 = Get Notifier Status(notifier=w478) -> (notifier out=w473:refnum<notifier>, current notification=w476:T13)  [unwired: 1 in, 3 out]
            n97 = Bundle By Name(cluster=w476, "Image Ref"=w475, "Action"=4Pi_4Pi_Modes_-_Mode_Scan_-_Scan_Actions."Exit") -> (w474:T13)
            n98 = Send Notification(notification=w474, notifier=w473) -> ()  [unwired: 1 in, 2 out]
          }
          event Value Change {
            n99 = event-data() -> ("NewVal"=w482:T6)  [unwired: 1 in]
            n100 = Get Notifier Status(notifier=w487) -> (notifier out=w484:refnum<notifier>, current notification=w486:T13)  [unwired: 1 in, 3 out]
            n101 = case shown="0, Default" w482 {
              tunnel: [T11."Enabled" ("Disabled") T11."Disabled and Grayed Out" ("Disabled")] -> w481
              frame 0, Default {
              }
              frame 1 {
              }
            }
            n102 = Bundle By Name(cluster=w486, "Fit Type"=w482, "Action"=4Pi_4Pi_Modes_-_Mode_Scan_-_Scan_Actions."Exit") -> (w485:T13)
            n103 = Send Notification(notification=w485, notifier=w484) -> ()  [unwired: 1 in, 2 out]
            n104 = property on="Gaussian Initial Guesses" class="Clust (strict)"("DisabledEnum"=w481) -> ()  [unwired: 2 in, 2 out]
          }
          event Value Change {
            w494 = T5 2 items=["Max Intensity", "No Zero Mean", "Threshold Mean", "Mean"] ("y")
            n105 = event-data() -> ("NewVal"=w495:T5)  [unwired: 1 in]
            n106 = Equal?(x=w495, y=w494) -> (x = y?=w493:bool)
            n107 = Get Notifier Status(notifier=w500) -> (notifier out=w498:refnum<notifier>, current notification=w499:T13)  [unwired: 1 in, 3 out]
            n108 = Bundle By Name(cluster=w499, "Metric"=w495, "Action"=4Pi_4Pi_Modes_-_Mode_Scan_-_Scan_Actions."Exit") -> (w497:T13)
            n109 = Select(t=T11."Enabled" ("Disabled"), s=w493, f=T11."Disabled and Grayed Out" ("Disabled")) -> (s? t:f=w490:T11)
            n110 = property on="Threshold Mean Limits" class="Clust (strict)"("DisabledEnum"=w490) -> ()  [unwired: 2 in, 2 out]
            n111 = Send Notification(notification=w497, notifier=w498) -> ()  [unwired: 1 in, 2 out]
          }
          event Value Change {
            w507 = T4 2 items=["Full Image", "ROI", "Blinks"] ("y")
            n112 = event-data() -> ("NewVal"=w508:T4)  [unwired: 1 in]
            n113 = Equal?(x=w508, y=w507) -> (x = y?=w502:bool)
            n114 = Get Notifier Status(notifier=w515) -> (notifier out=w513:refnum<notifier>, current notification=w514:T13)  [unwired: 1 in, 3 out]
            n115 = Bundle By Name(cluster=w514, "Image Type"=w508, "Action"=4Pi_4Pi_Modes_-_Mode_Scan_-_Scan_Actions."Exit") -> (w512:T13)
            n116 = Select(t=T11."Enabled" ("Disabled"), s=w502, f=T11."Disabled and Grayed Out" ("Disabled")) -> (s? t:f=w506:T11)
            n117 = Send Notification(notification=w512, notifier=w513) -> ()  [unwired: 1 in, 2 out]
            n118 = property on="Blink Scan Settings" class="Clust (strict)"("DisabledEnum"=w506) -> ()  [unwired: 2 in, 2 out]
            n119 = Select(t=T11."Disabled and Grayed Out" ("Disabled"), s=w502, f=T11."Enabled" ("Disabled")) -> (s? t:f=w503:T11)
            n120 = property on="Metric" class="Ring (strict)"("DisabledEnum"=w503) -> ()  [unwired: 2 in, 2 out]
          }
          event Value Change {
            n121 = event-data() -> ("NewVal"=w518:T2)  [unwired: 1 in]
            n122 = Get Notifier Status(notifier=w523) -> (notifier out=w520:refnum<notifier>, current notification=w522:T13)  [unwired: 1 in, 3 out]
            n123 = Bundle By Name(cluster=w522, "Gaussian Initial Guesses"=w518, "Action"=4Pi_4Pi_Modes_-_Mode_Scan_-_Scan_Actions."Exit") -> (w521:T13)
            n124 = Send Notification(notification=w521, notifier=w520) -> ()  [unwired: 1 in, 2 out]
          }
          event Value Change {
            n125 = event-data() -> ("NewVal"=w525:T3)  [unwired: 1 in]
            n126 = Get Notifier Status(notifier=w530) -> (notifier out=w527:refnum<notifier>, current notification=w529:T13)  [unwired: 1 in, 3 out]
            n127 = Bundle By Name(cluster=w529, "DM Scan Settings"=w525, "Action"=4Pi_4Pi_Modes_-_Mode_Scan_-_Scan_Actions."Exit") -> (w528:T13)
            n128 = Send Notification(notification=w528, notifier=w527) -> ()  [unwired: 1 in, 2 out]
          }
          event Value Change {
            n129 = event-data() -> ("NewVal"=w532:T7)  [unwired: 1 in]
            n130 = Get Notifier Status(notifier=w537) -> (notifier out=w534:refnum<notifier>, current notification=w536:T13)  [unwired: 1 in, 3 out]
            n131 = Bundle By Name(cluster=w536, "Threshold Mean Limits"=w532, "Action"=4Pi_4Pi_Modes_-_Mode_Scan_-_Scan_Actions."Exit") -> (w535:T13)
            n132 = Send Notification(notification=w535, notifier=w534) -> ()  [unwired: 1 in, 2 out]
          }
          event Value Change {
            n133 = event-data() -> ("NewVal"=w539:T8)  [unwired: 1 in]
            n134 = Get Notifier Status(notifier=w544) -> (notifier out=w541:refnum<notifier>, current notification=w543:T13)  [unwired: 1 in, 3 out]
            n135 = Bundle By Name(cluster=w543, "Blink Scan Settings"=w539, "Action"=4Pi_4Pi_Modes_-_Mode_Scan_-_Scan_Actions."Exit") -> (w542:T13)
            n136 = Send Notification(notification=w542, notifier=w541) -> ()  [unwired: 1 in, 2 out]
          }
          event "Exit": Value Change {
            n137 = event-data() -> ()  [unwired: 1 in, 1 out]
            n138 = Release Notifier(notifier=w551) -> ()  [unwired: 2 in, 3 out]
            n139 = Get Notifier Status(notifier=w549) -> (notifier out=w550:refnum<notifier>, current notification=w548:T13)  [unwired: 1 in, 3 out]
            n140 = Bundle By Name(cluster=w548, "Action"=4Pi_4Pi_Modes_-_Mode_Scan_-_Scan_Actions."Quit") -> (w547:T13)
            n141 = Send Notification(notification=w547, notifier=w550) -> ()  [unwired: 1 in, 2 out]
          }
        }
      }
      n142 = while {
        tunnel: w123 -> [w135]
        tunnel: w122 -> [w134]
        tunnel: w119 -> [w133]
        tunnel: w118 -> [w126]
        tunnel: [w126] -> w117
        stop <- w129 stop-if-true
        n143 = Wait on Notification(notifier=w133, ignore previous (F)=TRUE) -> (notifier out=w130:refnum<notifier>, notification=w131:T13)  [unwired: 2 in, 2 out]
        n144 = Unbundle By Name(w131) -> ("Action"=w127:T12)
        n145 = Equal?(x=4Pi_4Pi_Modes_-_Mode_Scan_-_Scan_Actions."Quit" ("y"), y=w127) -> (x = y?=w129:bool)
        n146 = while {
          shift-right: [w148] -> _
          shift-left: w127 -> [w142]
          tunnel: w135 -> [w147]
          tunnel: w134 -> [w146]
          tunnel: w130 -> [w145]
          tunnel: w126 -> [w140]
          shift-right: [w138] -> _
          shift-left: u16 0 -> [w139]
          shift-right: [w136] -> _
          shift-left: 0.0 -> [w137]
          stop <- w149 stop-if-true
          n147 = Get Notifier Status(notifier=w145) -> (notifier out=w144:refnum<notifier>, current notification=w143:T13)  [unwired: 1 in, 3 out]
          n148 = case shown="\"Apply Correction\"" w142 {
            selector: w142 -> [_ _ _ _ _ _ _ _ w402]
            tunnel: [w154 w169 w202 w259 w302 w310 w375 w393 TRUE] -> w149
            tunnel: [4Pi_4Pi_Modes_-_Mode_Scan_-_Scan_Actions."Update Mode Amount" ("y") 4Pi_4Pi_Modes_-_Mode_Scan_-_Scan_Actions."Get Image" ("y") w198 4Pi_4Pi_Modes_-_Mode_Scan_-_Scan_Actions."Update Counter" ("y") w303 4Pi_4Pi_Modes_-_Mode_Scan_-_Scan_Actions."Apply Correction" ("y") 4Pi_4Pi_Modes_-_Mode_Scan_-_Scan_Actions."Exit" ("y") 4Pi_4Pi_Modes_-_Mode_Scan_-_Scan_Actions."Scan Mode" ("y") 4Pi_4Pi_Modes_-_Mode_Scan_-_Scan_Actions."Exit" ("y")] -> w148
            tunnel: w147 -> [_ w174 _ _ _ _ w378 _ w400]
            tunnel: w146 -> [_ w172 w205 _ _ _ _ _ _]
            tunnel: w144 -> [_ _ _ _ _ _ _ _ w401]
            tunnel: w143 -> [w157 w170 w204 w263 _ w313 _ _ _]
            tunnel: FALSE -> [w154 w169 w202 w259 w302 w310 w375 w393 _]
            tunnel: w140 -> [_ _ w200 w258 _ _ _ _ _]
            tunnel: w139 -> [w153 w168 w197 w257 w301 w309 w374 w392 w399]
            tunnel: [w153 w168 w196 w257 w301 w309 w374 w392 w399] -> w138
            tunnel: w137 -> [w152 w167 w191 w255 w300 w308 w373 w391 w398]
            tunnel: [w152 w167 w190 w255 w300 w308 w373 w391 w398] -> w136
            frame "Scan Mode" {
              n149 = Unbundle By Name(w157) -> ("DM Scan Settings.Number of Steps"=w155:u16, "DM Scan Settings.Step Size (nm)"=w156:u16)
              n150 = call "4Pi 4Pi Modes - Coefficients  AE.vi"("Action"=4Pi_4Pi_Modes_-_Standard_Action."Read") -> ("Coefficients Out"=w150:cluster{"Mode":string, "Amplitude":dbl}[])  [unwired: 14 in]
              n151 = Initialize Array(0.0 ("element"), 0 ("dimension size")) -> (w160:dbl[])
              n152 = call "4Pi 4Pi Modes - Mode Scan Data AE.vi"("Amplitude"=w160, "Action"=4Pi_4Pi_Modes_-_Standard_Action."Write", "Metric"=w160) -> ()  [unwired: 11 in, 2 out]
              n153 = Index Array(array=w150, index="Current Mode") -> (element=w165:cluster{"Mode":string, "Amplitude":dbl})
              n154 = Unbundle By Name(w165) -> ("Amplitude"=w166:dbl)
              n155 = call "4Pi 4Pi Modes - Mode Scan Counter.vi"("Center Value"=w166, "Action"=4Pi_4Pi_Modes_-_Standard_Counter_Action."Initialize", "Mode"="Current Mode", "Number of Steps"=w155, "Step Size"=w156) -> ()  [unwired: 8 in, 3 out]
            }
            frame "Update Mode Amount" {
              n156 = flat-sequence {
                tunnel: w174 -> [w182]
                tunnel: [w182] -> w173
                tunnel: w173 -> [w185]
                tunnel: w172 -> [w189]
                tunnel: w170 -> [w188]
                frame #0 {
                  n157 = call "4Pi 4Pi Modes - Coefficients  AE.vi"("Action"=4Pi_4Pi_Modes_-_Standard_Action."Read") -> ("Coefficients Out"=w177:cluster{"Mode":string, "Amplitude":dbl}[])  [unwired: 14 in]
                  n158 = call "4Pi 4Pi Modes - Mode Scan Counter.vi"("Action"=4Pi_4Pi_Modes_-_Standard_Counter_Action."Get Count") -> ("Mode Amount"=w179:dbl, "Current Mode"=w180:i32)  [unwired: 12 in, 1 out]
                  n159 = Index Array(array=w177, index=w180) -> (element=w183:cluster{"Mode":string, "Amplitude":dbl})
                  n160 = Bundle By Name(cluster=w183, "Amplitude"=w179) -> (w184:cluster{"Mode":string, "Amplitude":dbl})
                  n161 = Replace Array Subset(array=w177, new element=w184, index=w180) -> (w175:cluster{"Mode":string, "Amplitude":dbl}[])
                  n162 = call "4Pi 4Pi Modes - Coefficients  AE.vi"("Coefficients In"=w175, "Action"=4Pi_4Pi_Modes_-_Standard_Action."Write") -> ()  [unwired: 13 in, 1 out]
                }
                frame #1 {
                  n163 = Enqueue Element(queue=w185, element="Mirror Modes" ("name (unnamed)")) -> ()  [unwired: 2 in, 3 out]
                }
                frame #2 {
                  n164 = Unbundle By Name(w188) -> ("DM Scan Settings.Frame Delay"=w187:u32)
                  n165 = call "4Pi 4Pi Modes - Confirm New Frame.vi"("Camera Notifier Name"=w189, "Wait No. (1)"=w187) -> ()  [unwired: 12 in, 2 out]
                }
              }
            }
            frame "Get Image" {
              n166 = Unbundle By Name(w204) -> ("Image Type"=w201:T4, "Image Ref"=w203:T1, "Blink Scan Settings.Blink Analysis Type"=w194:T9, "Blink Scan Settings.Blink Threshold"=w193:sgl, "Blink Scan Settings.Blink ROI Box Width"=w192:u8, "DM Scan Settings.Frame Accumulations"=w195:u16)
              n167 = case shown="2" w201 {
                tunnel: w205 -> [w211 w222 w247]
                tunnel: w203 -> [w210 w221 w245]
                tunnel: w195 -> [w208 w220 w254]
                tunnel: w200 -> [w209 w218 _]
                tunnel: [w207 w215 w229] -> w199
                tunnel: [4Pi_4Pi_Modes_-_Mode_Scan_-_Scan_Actions."Compute Metric" ("y") 4Pi_4Pi_Modes_-_Mode_Scan_-_Scan_Actions."Compute Metric" ("y") w248] -> w198
                tunnel: w197 -> [w212 w216 w228]
                tunnel: [w212 w216 w251] -> w196
                tunnel: w193 -> [_ _ w244]
                tunnel: w194 -> [_ _ w233]
                tunnel: w192 -> [_ _ w238]
                tunnel: w191 -> [w206 w214 w226]
                tunnel: [w206 w214 w227] -> w190
                frame 0, Default {
                  # "Full Image"
                  n168 = call "4Pi 4Pi Modes - Get Image Full.vi"("Camera Notifier Name"=w211, "Image Ref"=w210, "Image Dst"=w209, "Frame Accums."=w208) -> ("Image Dst Out"=w207:T1)  [unwired: 11 in]
                }
                frame 1 {
                  # "ROI"
                  n169 = call "4Pi 4Pi Modes - Get Image ROI.vi"("Camera Notifier Name"=w222, "Image Ref"=w221, "Frame Accums."=w220) -> ("Image Out"=w219:u16[][])  [unwired: 12 in]
                  n170 = call "IMAQ ArrayToImage"("Image Pixels (U16)"=w219, "Image"=w218) -> ("Image Out"=w215:T1)  [unwired: 8 in, 1 out]
                }
                frame 2 {
                  # "Blinks"
                  n171 = Increment(x=w228) -> (x+1=w252:u16)
                  n172 = Equal To 0?(x=w228) -> (x = 0?=w224:bool)
                  n173 = call "4Pi 4Pi Modes - Confirm New Frame.vi"("Camera Notifier Name"=w247, "Wait No. (1)"=u32 1) -> ("Error Out"=w243:errorcluster)  [unwired: 12 in, 1 out]
                  n174 = Greater Or Equal?(x=w252, y=w254) -> (x >= y?=w231:bool)
                  n175 = call "SMS Candidate Selection.vi"("Image Ref (U16)"=w245, "Blink Sensitivity"=w244, "Error In"=w243) -> ("Image Ref (U16) - Dup"=w229:T1, "Cadidate Image Ref"=w242:T1, "Error Out"=w241:errorcluster)  [unwired: 10 in]
                  n176 = Select(t=u16 0 ("f"), s=w231, f=w252) -> (s? t:f=w251:u16)
                  n177 = call "IMAQ DLL - Non Zero Indices.vi"("IMAQ Ref"=w242, "Error In"=w241) -> ("Row Column Indices"=w240:i32[][], "Error Out"=w239:errorcluster)  [unwired: 10 in, 2 out]
                  n178 = call "SMS Candidate Selection - Locations to ROIs.vi"("Image Ref"=w229, "Row Column Indices"=w240, "Error"=w239, "Box Half Size"=w238) -> ("Image Ref (DUP)"=w236:T1, "Image ROIs"=w237:T26, "ROI Coordinates (Left, Top, Right, Bottom)"=w235:i32[][], "Error Out"=w234:errorcluster)  [unwired: 8 in]
                  n179 = call "SMS Candidate Selection - Pull Sub Regions.vi"("Image Ref"=w236, "ROI Coordinates"=w235, "Error"=w234) -> ("ROIs"=w232:u16[][][])  [unwired: 10 in, 2 out]
                  n180 = property on="AO Image Display" class="ImageControl"("ROI"=w237) -> ()  [unwired: 2 in, 2 out]
                  n181 = Select(t=0.0, s=w224, f=w226) -> (s? t:f=w223:dbl)
                  n182 = call "4Pi 4Pi Modes - Fit Sum ROIs.vi"("Blink Analysis Type"=w233, "ROIs"=w232) -> ("Blink Metric"=w225:dbl)  [unwired: 13 in]
                  n183 = Add(x=w225, y=w223) -> (x+y=w227:dbl)
                  n184 = Select(t=4Pi_4Pi_Modes_-_Mode_Scan_-_Scan_Actions."Compute Metric" ("y"), s=w231, f=4Pi_4Pi_Modes_-_Mode_Scan_-_Scan_Actions."Get Image") -> (s? t:f=w248:T12)
                }
              }
              "AO Image Display" <- w199
            }
            frame "Compute Metric" {
              n185 = Unbundle By Name(w263) -> ("Image Type"=w256:T4, "Metric"=w262:T5, "Threshold Mean Limits.Upper Limit"=w261:dbl, "Threshold Mean Limits.Lower Limit"=w260:dbl)
              n186 = case shown="Default" w256 {
                tunnel: [w282 w299] -> w270
                tunnel: w262 -> [w280 _]
                tunnel: w261 -> [w279 _]
                tunnel: w260 -> [w278 _]
                tunnel: w258 -> [w277 _]
                tunnel: w255 -> [_ w299]
                frame Default {
                  n187 = call "IMAQ ImageToArray"("Image"=w277) -> ("Image Pixels (U16)"=w276:u16[][])  [unwired: 3 in, 4 out]
                  n188 = To Double Precision Float(number=w276) -> (double precision float=w281:dbl[][])
                  n189 = case shown="3" w280 {
                    tunnel: w281 -> [w285 w288 w293 w297]
                    tunnel: [w283 w287 w291 w294] -> w282
                    tunnel: w279 -> [_ _ w290 _]
                    tunnel: w278 -> [_ _ w289 _]
                    frame 0, Default {
                      # "Max Pixel Value"
                      n190 = Array Max & Min(array=w285) -> (max value=w284:dbl)  [unwired: 3 out]
                      n191 = To Double Precision Float(number=w284) -> (double precision float=w283:dbl)
                    }
                    frame 1 {
                      # "No Zero Mean"
                      n192 = call "4Pi 4Pi Modes - No Zeros Mean.vi"("Image IN"=w288, "STDev Factor"=0.0) -> ("No Zero Mean"=w287:dbl)  [unwired: 13 in]
                    }
                    frame 2 {
                      # "Threshold Array Mean"
                      n193 = call "4Pi 4Pi Modes - Threshold 2D Array.vi"("2D Array IN"=w293, "Upper Limit"=w290, "Lower Limit"=w289) -> ("Threshold Array Out"=w292:dbl[])  [unwired: 12 in]
                      n194 = call-poly <vilib>:"Mean.vi"("X"=w292) -> ("mean"=w291:dbl)  [unwired: 1 out]
                    }
                    frame 3 {
                      # "Mean"
                      n195 = Array Size(array=w297) -> (size(s)=w298:i32[])
                      n196 = Multiply Array Elements(1:w298) -> (0:w296:i32)
                      n197 = Reshape Array(w297, w296) -> (w295:dbl[])
                      n198 = call-poly <vilib>:"Mean.vi"("X"=w295) -> ("mean"=w294:dbl)  [unwired: 1 out]
                    }
                  }
                }
                frame 2 {
                }
              }
              n199 = call "4Pi 4Pi Modes - Mode Scan Data AE.vi"("Action"=4Pi_4Pi_Modes_-_Standard_Action."Read") -> ("Amplitude Out"=w267:dbl[], "Metric Out"=w268:dbl[])  [unwired: 13 in]
              n200 = call "4Pi 4Pi Modes - Mode Scan Counter.vi"("Action"=4Pi_4Pi_Modes_-_Standard_Counter_Action."Get Count") -> ("Mode Amount"=w269:dbl)  [unwired: 12 in, 2 out]
              n201 = Build Array (concatenate)(w268, w270) -> (w273:dbl[])
              n202 = Build Array (concatenate)(w267, w269) -> (w272:dbl[])
              n203 = call "4Pi 4Pi Modes - Mode Scan Data AE.vi"("Amplitude"=w272, "Action"=4Pi_4Pi_Modes_-_Standard_Action."Write", "Metric"=w273) -> ()  [unwired: 11 in, 2 out]
              n204 = Bundle(w272, w273) -> (w274:cluster{dbl[], dbl[]})  [unwired: 1 in]
              n205 = Build Array(w274) -> (→"Metric":cluster{dbl[], dbl[]}[])
            }
            frame "Update Counter" {
              n206 = call "4Pi 4Pi Modes - Mode Scan Counter.vi"("Action"=4Pi_4Pi_Modes_-_Standard_Counter_Action."Update Count") -> ("Scan Done?"=w306:bool)  [unwired: 12 in, 2 out]
              n207 = Select(t=4Pi_4Pi_Modes_-_Mode_Scan_-_Scan_Actions."Fit Data" ("y"), s=w306, f=4Pi_4Pi_Modes_-_Mode_Scan_-_Scan_Actions."Update Mode Amount" ("y")) -> (s? t:f=w303:T12)
            }
            frame "Fit Data" {
              n208 = Unbundle By Name(w313) -> ("Gaussian Initial Guesses"=w312:T2, "Fit Type"=w311:T6)
              n209 = call "4Pi 4Pi Modes - Mode Scan Data AE.vi"("Action"=4Pi_4Pi_Modes_-_Standard_Action."Read") -> ("Amplitude Out"=w323:dbl[], "Metric Out"=w324:dbl[])  [unwired: 13 in]
              n210 = Bundle("Amplitude Out"=w323, "Metric Out"=w324) -> (w322:T27)  [unwired: 1 in]
              n211 = case shown="1" w311 {
                tunnel: w323 -> [w328 w372]
                tunnel: w324 -> [w356 w371]
                tunnel: [w347 w368] -> w317
                tunnel: [w346 w369] -> w320
                tunnel: [w345 w370] -> w319
                tunnel: w312 -> [w343 _]
                frame 0, Default {
                  n212 = To Double Precision Float(number=w356) -> (double precision float=w355:dbl[])
                  n213 = Array Max & Min(array=w328) -> (max value=w334:dbl, min value=w333:dbl)  [unwired: 2 out]
                  n214 = Unbundle By Name(w343) -> ("Amplitude"=w342:dbl, "Center Position"=w341:dbl, "Width (Sigma)"=w340:dbl, "Offset"=w339:dbl, "User Guesses"=w326:bool)
                  n215 = Array Max & Min(array=w355) -> (max value=w336:dbl, max index (indices)=w329:i32, min value=w335:dbl)  [unwired: 1 out]
                  n216 = Subtract(x=w334, y=w333) -> (x-y=w332:dbl)
                  n217 = Divide(x=w332, y=2.0) -> (x/y=w330:dbl)
                  n218 = Bundle By Name(cluster=T23 {"initial amplitude"=nan, "initial center"=nan, "initial standard deviation"=nan, "offset"=nan} ("initial guess"), "initial amplitude"=w342, "initial center"=w341, "initial standard deviation"=w340, "offset"=w339) -> (w337:T23)
                  n219 = Index Array(array=w328, index=w329) -> (element=w327:dbl)
                  n220 = Bundle(w336, "Numeric"=w327, w330, w335) -> (w354:cluster{dbl, "Numeric":dbl, dbl, dbl})  [unwired: 1 in]
                  n221 = Select(t=w337, s=w326, f=w354) -> (s? t:f=w338:T28)
                  n222 = call <vilib>:"Gaussian Peak Fit.vi"("Y"=w355, "initial guess"=w338, "X"=w328, "parameter bounds"=T24 {"amp min"=0.0, "amp max"=100000.0, "center min"=-100.0, "center max"=100.0, "deviation min"=0.0, "deviation max"=1000.0, "offset min"=0.0, "offset max"=1000.0}) -> ("offset"=w350:dbl, "amplitude"=w352:dbl, "center"=w347:dbl, "standard deviation"=w351:dbl)  [unwired: 5 in, 3 out]
                  n223 = Build Array(w352, w347, w351, w350) -> (w349:dbl[])
                  n224 = call "4Pi 4Pi Modes - 1D Gaussian.vi"("Parameters In"=w349, "Number of Points"=1000.0, "Max X Value"=w334, "Min X Value"=w333) -> ("X Values"=w346:dbl[], "Y Values"=w345:dbl[])  [unwired: 10 in]
                }
                frame 1 {
                  w366 = T29 2 items=["Least Square", "Least Absolute Residual", "Bisquare"] ("method")
                  # "LV often can't find this file. It should be located at C:\\Program Files\\National Instruments\\LabVIEW 2016\\examples\\Mathematics\\Fitting\\support"
                  n225 = To Double Precision Float(number=w371) -> (double precision float=w367:dbl[])
                  n226 = call <vilib>:"General Polynomial Fit.vi"("Y"=w367, "polynomial order"=2, "X"=w372, "method"=w366) -> ("Polynomial Coefficients"=w363:dbl[])  [unwired: 8 in, 3 out]
                  n227 = Array Max & Min(array=w372) -> (max value=w359:dbl, min value=w358:dbl)  [unwired: 2 out]
                  n228 = call "NI- Regression Equation String.vi"("coefficients"=w363, "precision"=3, "fit type"=T25."Polynomial") -> ("Formula"=w361:string)  [unwired: 8 in]
                  n229 = call <vilib>:"Eval y=f(x) Optimal Step.vi"("number of points"=u32 3000, "formula"=w361, "end"=w359, "start"=w358) -> ("Y Values"=w370:dbl[], "X Values"=w369:dbl[])  [unwired: 1 in, 2 out]
                  n230 = Array Max & Min(array=w370) -> (max index (indices)=w357:i32)  [unwired: 3 out]
                  n231 = Index Array(array=w369, index=w357) -> (element=w368:dbl)
                }
              }
              n232 = Bundle("X Values"=w320, "Y Values"=w319) -> (w318:cluster{"X Values":dbl[], "Y Values":dbl[]})  [unwired: 1 in]
              n233 = Build Array(w322, w318) -> (w321:cluster{"X Values":dbl[], "Y Values":dbl[]}[])
              n234 = property on="Metric" class="XYGraph (strict)"("Cursor.Cursor X"=w317, "Cursor.Cursor Y"=-10000.0 ("Cursor.Cursor Position:Cursor X"), "Cursor.Visible"=TRUE, "Value"=w321) -> ()  [unwired: 2 in, 2 out]
            }
            frame "Apply Correction" {
              n235 = flat-sequence {
                tunnel: w378 -> [w388]
                tunnel: [w388] -> w377
                tunnel: w377 -> [w389]
                frame #0 {
                  n236 = call "4Pi 4Pi Modes - Coefficients  AE.vi"("Action"=4Pi_4Pi_Modes_-_Standard_Action."Read") -> ("Coefficients Out"=w379:cluster{"Mode":string, "Amplitude":dbl}[])  [unwired: 14 in]
                  n237 = property on="Metric" class="XYGraph (strict)"() -> ("Cursor.Cursor X"=w387:dbl)  [unwired: 2 in, 2 out]
                  n238 = call "4Pi 4Pi Modes - Mode Scan Counter.vi"("Action"=4Pi_4Pi_Modes_-_Standard_Counter_Action."Get Count") -> ("Current Mode"=w386:i32)  [unwired: 12 in, 2 out]
                  n239 = Index Array(array=w379, index=w386) -> (element=w384:cluster{"Mode":string, "Amplitude":dbl})
                  n240 = Bundle By Name(cluster=w384, "Amplitude"=w387) -> (w383:cluster{"Mode":string, "Amplitude":dbl})
                  n241 = Replace Array Subset(array=w379, new element=w383, index=w386) -> (w381:cluster{"Mode":string, "Amplitude":dbl}[])
                  n242 = call "4Pi 4Pi Modes - Coefficients  AE.vi"("Coefficients In"=w381, "Action"=4Pi_4Pi_Modes_-_Standard_Action."Write") -> ()  [unwired: 13 in, 1 out]
                }
                frame #1 {
                  n243 = Enqueue Element(queue=w389, element="Mirror Modes" ("name (unnamed)")) -> ()  [unwired: 2 in, 3 out]
                }
              }
            }
            frame "Scan Next Mode" {
              n244 = call "4Pi 4Pi Modes - Mode Scan Counter.vi"("Action"=4Pi_4Pi_Modes_-_Standard_Counter_Action."Get Count") -> ("Current Mode"=w396:i32)  [unwired: 12 in, 2 out]
              n245 = Increment(x=w396) -> (x+1=w397:i32)
              n246 = local write "Current Mode"(w397) -> ()
            }
            frame "Exit", "Quit" {
              n247 = case shown="\"Quit\"" w402 {
                tunnel: w401 -> [w423 _]
                tunnel: w400 -> [w424 _]
                frame "Quit" {
                  w421 = T14 {"Image Ref Index"=0, "Image Type"=0, "Fit Type"=0, "Metric"=1, "DM Scan Settings"={"Frame Delay"=1, "Frame Accumulations"=2, "Number of Steps"=8, "Step Size (nm)"=80}, "Threshold Mean Limits"={"Upper Limit"=10000.0, "Lower Limit"=0.0}, "Gaussian Initial Guesses"={"Amplitude"=2500.0, "Center Position"=0.0, "Width (Sigma)"=200.0, "Offset"=500.0, "User Guesses"=TRUE}, "Blink Scan Settings"={"Blink Analysis Type"=1, "Blink ROI Box Width"=0, "Blink Threshold"=0.0}}  # Last Used Scan Settings
                  n248 = Release Notifier(notifier=w423, force destroy? (F)=TRUE) -> (last notification=w422:T13)  [unwired: 1 in, 2 out]
                  n249 = Release Queue(queue=w424) -> ()  [unwired: 2 in, 3 out]
                  n250 = Unbundle By Name(w422) -> ("Image Type"=w420:T4, "Fit Type"=w418:T6, "Metric"=w417:T5, "DM Scan Settings"=w416:T3, "Threshold Mean Limits"=w415:T7, "Gaussian Initial Guesses"=w414:T2, "Blink Scan Settings"=w413:T8)
                  n251 = local read "Image Selection"() -> (w419:i32)
                  n252 = control-ref of="This VI"() -> (w412:refnum<vi>)
                  n253 = property class="VI"(reference=w412) -> ("Path"=w411:path)  [unwired: 1 in, 2 out]
                  n254 = Bundle By Name(cluster=w421, "Image Ref Index"=w419, "Image Type"=w420, "Fit Type"=w418, "Metric"=w417, "DM Scan Settings"=w416, "Threshold Mean Limits"=w415, "Gaussian Initial Guesses"=w414, "Blink Scan Settings"=w413) -> (w407:T14)
                  n255 = Strip Path(path=w411) -> (stripped path=w410:path)  [unwired: 1 out]
                  n256 = Strip Path(path=w410) -> (stripped path=w409:path)  [unwired: 1 out]
                  n257 = Build Path(base path=w409, name or relative path="4Pi Dual DM - Default Files\\Last Used Scan Settings.json") -> (appended path=w405:path)
                  n258 = Flatten To JSON(anything=w407) -> (JSON string=w406:string)  [unwired: 2 in, 1 out]
                  n259 = Write to Text File(file (use dialog)=w405, text=w406) -> ()  [unwired: 2 in, 3 out]
                }
                frame "Exit", Default {
                }
              }
            }
          }
        }
      }
      n260 = call "IMAQ Dispose"("Image"=w117) -> ()  [unwired: 5 in, 1 out]
    }
    frame Error {
      n261 = Release Notifier(notifier=w552) -> ()  [unwired: 2 in, 3 out]
      n262 = Release Notifier(notifier=w553) -> ()  [unwired: 2 in, 3 out]
      n263 = Release Queue(queue=w554) -> ()  [unwired: 2 in, 3 out]
      n264 = call "IMAQ Dispose"("Image"=w555) -> ()  [unwired: 5 in, 1 out]
    }
  }
